vi "StateMachine.vi"() -> ()   [LabVIEW 2023]
uses:
  TypeDef.ctl
panel:
  out "통신":bool
  out "분석":bool
  out "측정":bool
  in  "stop":bool
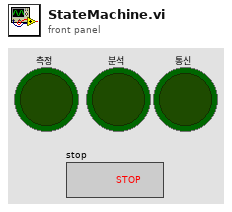
[diagram p1: front panel]
types:
  T1 = typedef "TypeDef.ctl" = enum16{"측정", "분석", "통신"}
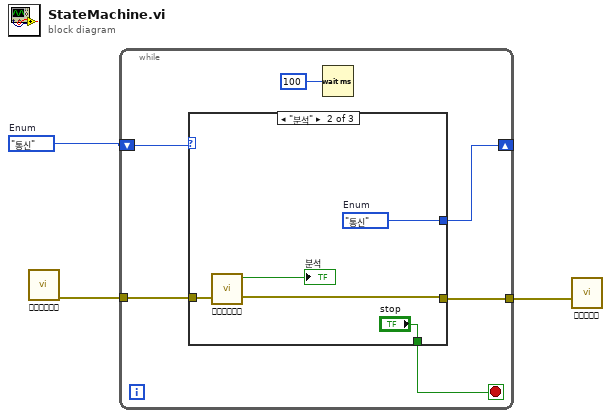
[diagram p0: block diagram]
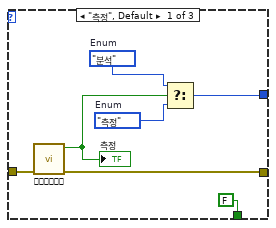
[diagram p2: hidden frame]
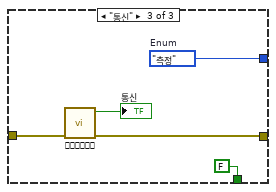
[diagram p3: hidden frame]
diagram:
  w1 = TypeDef."통신"  # Enum
  n1 = call "설정.vi"() -> ("error out"=w3:errorcluster)  [unwired: 11 in]
  n2 = while {
    tunnel: w3 -> [w8]
    tunnel: [w7] -> w2
    shift-right: [w5] -> _
    shift-left: w1 -> [w4]
    stop <- w6 stop-if-true
    n3 = case shown="\"분석\"" w4 {
      tunnel: w8 -> [w16 w21 w25]
      tunnel: [w15 w20 w24] -> w7
      tunnel: [w14 w18 w22] -> w5
      tunnel: [FALSE ("stop") "stop" FALSE ("stop")] -> w6
      frame "측정", Default {
        w10 = TypeDef."측정"  # Enum
        w11 = TypeDef."분석"  # Enum
        n4 = call "측정.vi"("error in"=w16) -> ("error out"=w15:errorcluster, "Boolean"=w13:bool)  [unwired: 9 in]
        "측정" <- w13
        n5 = Select(t=w11, s=w13, f=w10) -> (s? t:f=w14:T1)
      }
      frame "분석" {
        w18 = TypeDef."통신"  # Enum
        n6 = call "분석.vi"("error in"=w21) -> ("error out"=w20:errorcluster, "Boolean"=→"분석":bool)  [unwired: 9 in]
      }
      frame "통신" {
        w22 = TypeDef."측정"  # Enum
        n7 = call "통신.vi"("error in"=w25) -> ("error out"=w24:errorcluster, "Boolean"=→"통신":bool)  [unwired: 9 in]
      }
    }
    n8 = Wait (ms)(milliseconds to wait=u32 100) -> ()  [unwired: 1 out]
  }
  n9 = call "종료.vi"("error in"=w2) -> ()  [unwired: 10 in, 1 out]
